vi "Query Table.vi"(8 "error in (no error)":errorcluster, 9 "Optional Clause":string, 10 "Table":string, 11 "connection reference":T1) -> (0 "error out":errorcluster, 2 "Data Output Array":string[][](array[string]), 3 "Column Names":string[](array[string]), 5 "connection reference out":T1)   [LabVIEW 2009]
uses:
  <vilib>/addons/database/Connection.llb/Conn ObjectReference.ctl
  <vilib>/addons/database/_DB Variant To Data/Database Variant To Data.xnode
  <vilib>/addons/database/NI_Database_API.lvlib
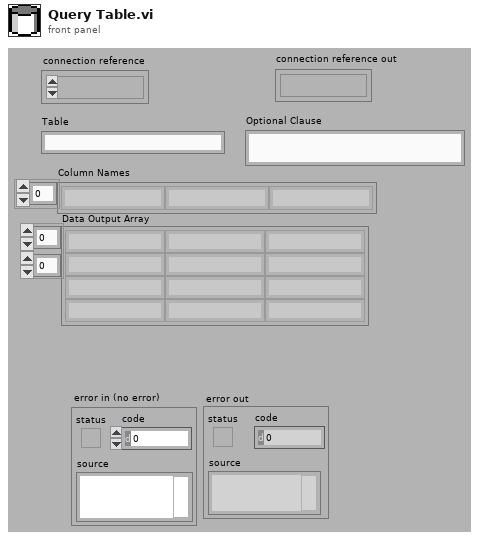
[diagram p1: front panel]
types:
  T1 = typedef "NI_Database_API.lvlib/Conn ObjectReference.ctl" = refnum<k1>
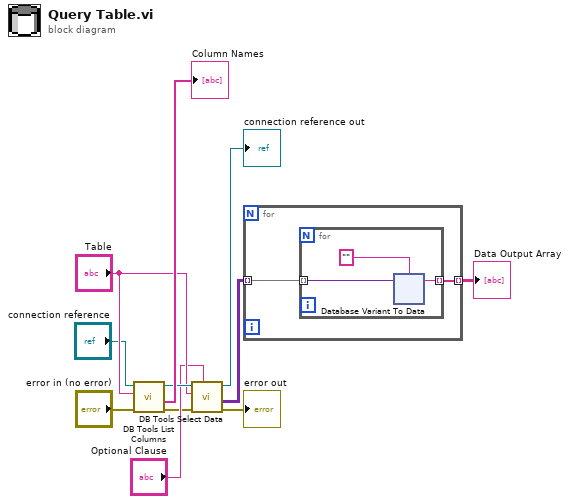
[diagram p0: block diagram]
diagram:
  n1 = call <vilib>:"DB Tools List Columns.vi"("error in (no error)"="error in (no error)", "table"="Table", "connection reference"="connection reference") -> ("error out"=w4:errorcluster, "columns"=→"Column Names":string[], "connection reference out"=w7:T1)  [unwired: 1 in, 1 out]
  n2 = call <vilib>:"DB Tools Select Data.vi"("optional clause"="Optional Clause", "error in (no error)"=w4, "table"="Table", "connection reference"=w7) -> ("error out"=→"error out":errorcluster, "data"=w9:variant[][], "connection reference out"=→"connection reference out":T1)  [unwired: 2 in]
  n3 = for {
    tunnel: w9 -> [w13] mode=indexing
    tunnel: [w12] -> w8 mode=indexing
    n4 = for {
      tunnel: w13 -> [w16] mode=indexing
      tunnel: [w14] -> w12 mode=indexing
      n5 = xnode "Database Variant To Data"("database variant"=w16, "type"="") -> ("data"=w14:string)  [unwired: 1 in, 1 out]
    }
  }
  "Data Output Array" <- w8
